vi "Read Bool.vi"(2 "Network Path":string, 5 "Tag Name":string) -> (1 "BOOL":bool)   [LabVIEW 2020]
uses:
  <vilib>/ethernetip/ethernetip.llb/EthernetIP Tag Read BOOL.vi
  <vilib>/ethernetip/ethernetip.lvlib
panel:
  out "error out":errorcluster
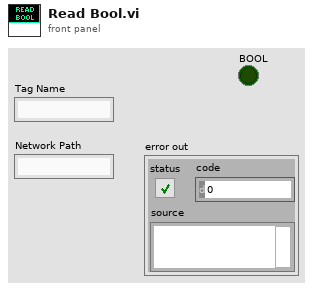
[diagram p1: front panel]
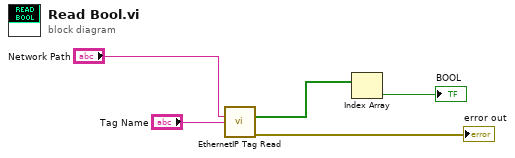
[diagram p0: block diagram]
diagram:
  n1 = call-poly <vilib>:"EthernetIP Tag Read.vi"("Network Path"="Network Path", "Tag Name"="Tag Name") -> ("Data"=w2:bool[], "error out"=→"error out":errorcluster)  [unwired: 3 in, 9 out]
  n2 = Index Array(array=w2) -> (element=→"BOOL":bool)  [unwired: 1 in]
